vi "Get Server gRPC UEs.vi"(11 "OOP Server in":refnum<class "server1.lvclass">) -> (2 "Server gRPC UEs":T1, 3 "OOP Server out":refnum<class "server1.lvclass">)   [LabVIEW 2020, in "server1.lvlib" / "server1.lvclass"]
uses:
  server1.lvclass
  typeDefs/Server gRPC UEs.ctl
  server1.lvclass/server1.ctl
  gRPC lvSupport/Server API/typeDefs/grpcId.ctl
  gRPC lvSupport/gprc-lvsupport.lvlib
  gRPC lvSupport/Server API/typeDefs/gRPCId Cluster.ctl
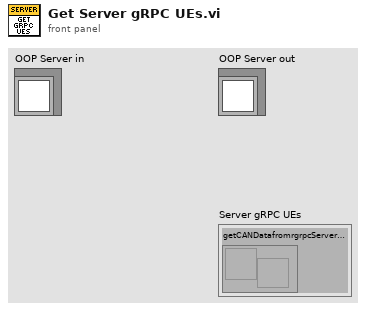
[diagram p1: front panel]
types:
  T1 = typedef "server1.lvlib/server1.lvclass/Server gRPC UEs.ctl" = cluster{"getCANDatafromrgrpcServer_clientRequester_getIDFormServer gRPC UE":refnum<user-event>}
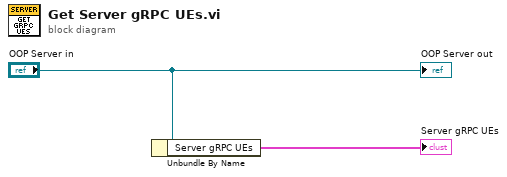
[diagram p0: block diagram]
diagram:
  n1 = Unbundle By Name("OOP Server in") -> ("Server gRPC UEs"=→"Server gRPC UEs":T1)
  "OOP Server out" <- "OOP Server in"
